vi "List Open FP in Project.vi"() -> (2 "FP refs":refnum<vi>[](array[refnum]), 3 "Open FPs":string[](array[string]))   [LabVIEW 2012]
uses:
  <userlib>/_OpenG.lib/array/array.llb/Conditional Auto-Indexing Tunnel (VI-REF)__ogtk.vi
  <userlib>/_OpenG.lib/array/array.llb/Conditional Auto-Indexing Tunnel (String)__ogtk.vi
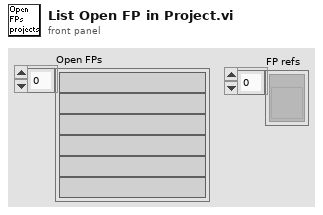
[diagram p1: front panel]
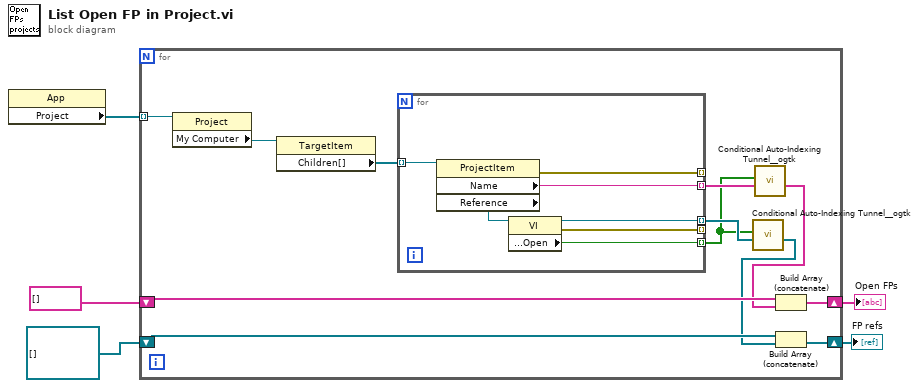
[diagram p0: block diagram]
diagram:
  n1 = property class="App"() -> ("Project"=w5:refnum<vi>[])  [unwired: 2 in, 2 out]
  n2 = for {
    tunnel: w5 -> [w14] mode=indexing
    shift-right: [w11] -> w4
    shift-left: string[] [] ("Array") -> [w13]
    shift-right: [w9] -> w2
    shift-left: refnum<vi>[] [] ("FP refs") -> [w10]
    n3 = property class="Project"(reference=w14) -> ("My Computer"=w17:refnum<vi>)  [unwired: 1 in, 2 out]
    n4 = property class="TargetItem"(reference=w17) -> ("Children[]"=w16:refnum<vi>[])  [unwired: 1 in, 2 out]
    n5 = for {
      tunnel: w16 -> [w24] mode=indexing
      tunnel: [w23] -> w15 mode=indexing
      tunnel: [w22] -> _ mode=indexing
      tunnel: [w20] -> w7 mode=indexing
      tunnel: [w19] -> _ mode=indexing
      tunnel: [w18] -> w8 mode=indexing
      n6 = property class="ProjectItem"(reference=w24) -> (error out=w22:errorcluster, "Name"=w23:string, "Reference"=w21:refnum<vi>)  [unwired: 1 in, 1 out]
      n7 = property class="VI"(reference=w21) -> (reference out=w18:refnum<vi>, error out=w19:errorcluster, "Front Panel.Open"=w20:bool)  [unwired: 1 in]
    }
    n8 = call-poly <userlib>:"Conditional Auto-Indexing Tunnel__ogtk.vi"("Array in"=w8, "Elements to keep"=w7) -> ("Filtered Array out"=w6:refnum<vi>[])  [unwired: 5 out]
    n9 = call-poly <userlib>:"Conditional Auto-Indexing Tunnel__ogtk.vi"("Array in"=w15, "Elements to keep"=w7) -> ("Filtered Array out"=w12:string[])  [unwired: 5 out]
    n10 = Build Array (concatenate)(w13, w12) -> (w11:string[])
    n11 = Build Array (concatenate)(w10, w6) -> (w9:refnum<vi>[])
  }
  "Open FPs" <- w4
  "FP refs" <- w2
